vi "CRYGet IOChannel Name.vi"(2 "O_Channel Info In":T1[](array[typedef]) {"Coupling" items=["Default"=-1, "RSE"=10083, "NRSE"=10078, "Differential"=10106, "Pseudodifferential"=12529]; "term config" items=["Default"=-1, "RSE"=10083, "NRSE"=10078, "Differential"=10106, "Pseudodifferential"=12529]; "Anti-aliasing Factor (%fs)" format="%.2f"}, 3 "I_Channel Info In":T1[](array[typedef]) {"Coupling" items=["Default"=-1, "RSE"=10083, "NRSE"=10078, "Differential"=10106, "Pseudodifferential"=12529]; "term config" items=["Default"=-1, "RSE"=10083, "NRSE"=10078, "Differential"=10106, "Pseudodifferential"=12529]; "Anti-aliasing Factor (%fs)" format="%.2f"}) -> (9 "O_Name Out":string[][](array[string]), 10 "I_Name Out":string[][](array[string]))   [LabVIEW 2013]
uses:
  Typedef Control/CRYHardware Channel Info.ctl
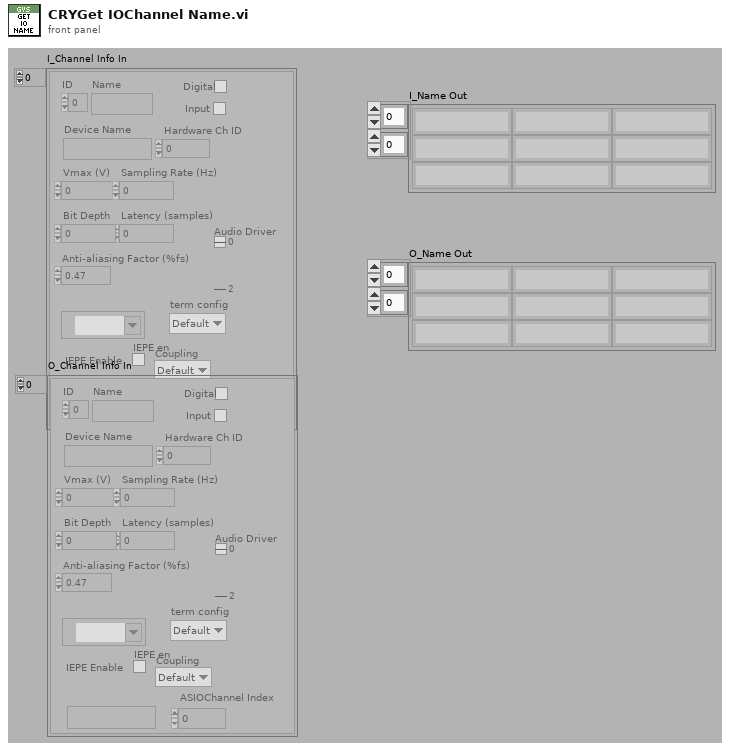
[diagram p1: front panel]
types:
  T1 = typedef "CRYHardware Channel Info.ctl" = cluster{"ID":i32, "Name":string, "Digital":bool, "Input":bool, "Device Name":string, "Hardware Ch ID":u8, "Vmax (V)":dbl, "Latency (samples)":dbl, "Sampling Rate (Hz)":u32, "Bit Depth":u32, "Anti-aliasing Factor (%fs)":sgl, "DAQmx Channel":tag, "term config":i32, "Coupling":i32, "IEPE en":bool, "ASIOChannel Name":string, "Audio Driver":u16, "ASIOChannel Index":u8}
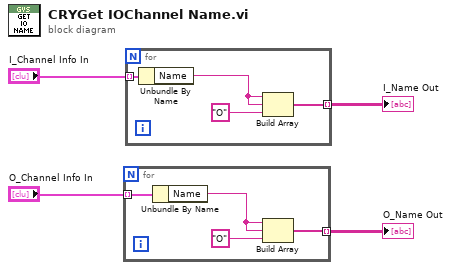
[diagram p0: block diagram]
diagram:
  n1 = for {
    tunnel: "O_Channel Info In" -> [w8] mode=indexing
    tunnel: [w6] -> w1 mode=indexing
    n2 = Unbundle By Name(w8) -> ("Name"=w5:string)
    n3 = Build Array(w5, w5, "O" ("Name")) -> (w6:string[])
  }
  "O_Name Out" <- w1
  n4 = for {
    tunnel: [w11] -> w3 mode=indexing
    tunnel: "I_Channel Info In" -> [w10] mode=indexing
    n5 = Unbundle By Name(w10) -> ("Name"=w9:string)
    n6 = Build Array(w9, w9, "O" ("Name")) -> (w11:string[])
  }
  "I_Name Out" <- w3
